vi "Init DAQ Analog In.vi"(8 "error in":errorcluster, 10 "name to assign":string, 11 "physical channels":tag="Dev1/ai0") -> (0 "error out":errorcluster, 3 "Refnum out":refnum<k21>)   [LabVIEW 2021]
uses:
  <vilib>/DAQmx/create/channels.llb/DAQmx Create Channel (AI-Voltage-Basic).vi
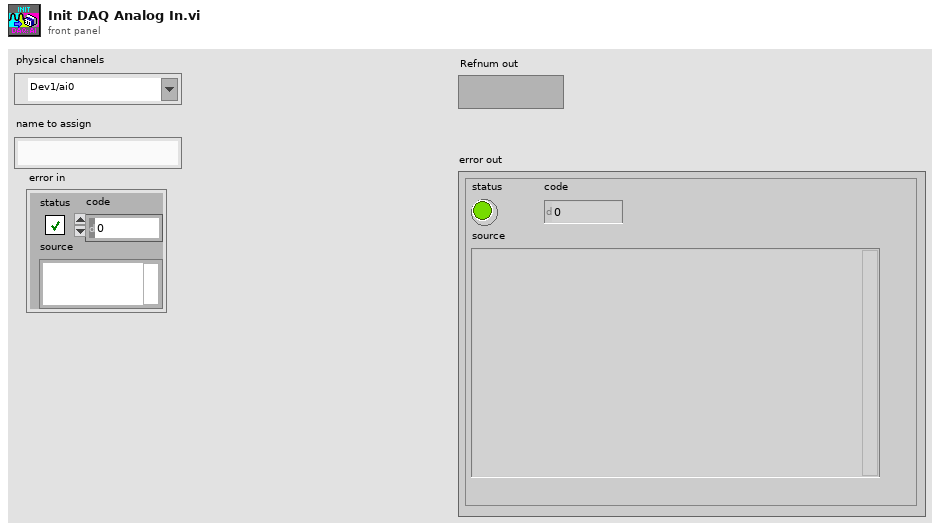
[diagram p1: front panel]
types:
  T1 = cluster{"first electrical value":dbl, "second electrical value":dbl, "electrical units":i32, "first physical value":dbl, "second physical value":dbl, "physical units":i32}
  T2 = cluster{"bridge configuration":i32, "voltage excitation source":i32, "voltage excitation value":dbl, "nominal bridge resistance":dbl}
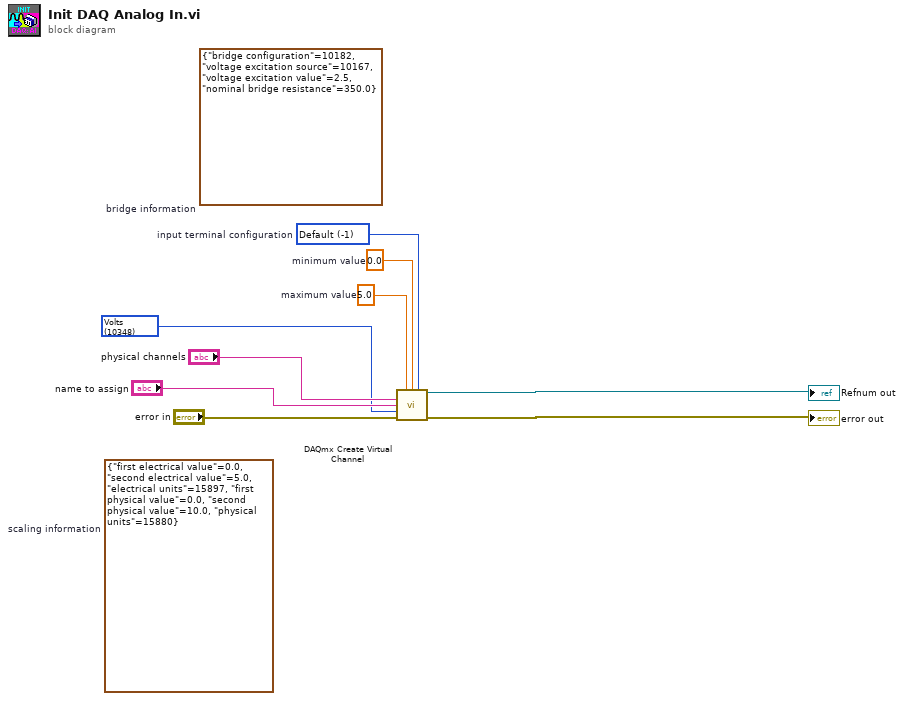
[diagram p0: block diagram]
diagram:
  w1 = 10348 items=["Volts"=10348, "From Custom Scale"=10065] ("units")
  w4 = -1 items=["Default"=-1, "RSE"=10083, "NRSE"=10078, "Differential"=10106, "Pseudodifferential"=12529]  # input terminal configuration
  (unwired) T1 {"first electrical value"=0.0, "second electrical value"=5.0, "electrical units"=15897, "first physical value"=0.0, "second physical value"=10.0, "physical units"=15880}  # scaling information
  (unwired) T2 {"bridge configuration"=10182, "voltage excitation source"=10167, "voltage excitation value"=2.5, "nominal bridge resistance"=350.0}  # bridge information
  w6 = 5.0  # maximum value
  w7 = 0.0  # minimum value
  n1 = call-poly <vilib>:"DAQmx Create Virtual Channel.vi"("maximum value"=w6, "minimum value"=w7, "input terminal configuration"=w4, "physical channels"="physical channels", "name to assign"="name to assign", "units"=w1, "error in"="error in") -> ("task out"=→"Refnum out":refnum<k21>, "error out"=→"error out":errorcluster)  [unwired: 7 in]
